vi "scale-percent-to-mA.vi"(11 "input %":dbl[](array[numeric])) -> (3 "Output mA":dbl[](array[numeric]))   [LabVIEW 2024]
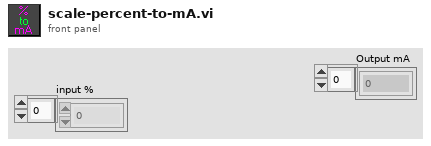
[diagram p1: front panel]
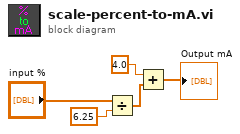
[diagram p0: block diagram]
diagram:
  n1 = Divide(x="input %", y=6.25 ("Pump 9")) -> (x/y=w4:dbl[])
  n2 = Add(x=4.0 ("Pump 9"), y=w4) -> (x+y=→"Output mA":dbl[])
